vi "Cleanup.vi"(8 "error in (no error)":errorcluster, 11 "Websocket Server in":refnum<class "Websocket Server.lvclass">) -> (0 "error out":errorcluster)   [LabVIEW 2020, in "Stream-Websocket.lvlib" / "Websocket Server.lvclass"]
uses:
  Websocket Server.lvclass
  C:/dev/lv20CE/relink/lv-stream/stream/Endpoint/Endpoint.lvclass
  Websocket Server.lvclass/Websocket Server.ctl
  lv-stream/stream/Endpoint/Endpoint.lvclass
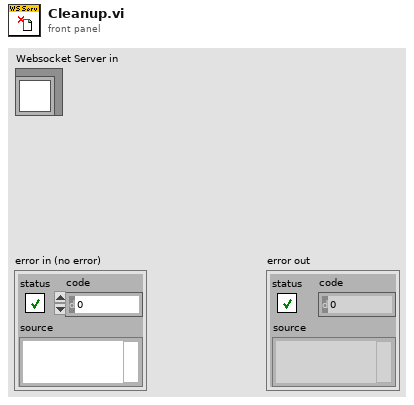
[diagram p1: front panel]
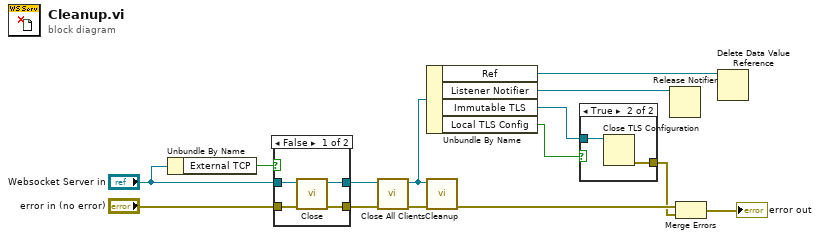
[diagram p0: block diagram]
diagram:
  n1 = Unbundle By Name("Websocket Server in") -> ("External TCP"=w2:bool)
  n2 = case shown="False" w2 {
    tunnel: "error in (no error)" -> [w18 w19]
    tunnel: [w17 w20] -> w12
    tunnel: [w16 w19] -> w11
    tunnel: "Websocket Server in" -> [w15 w20]
    frame False {
      n3 = call "Close.vi"("error in (no error)"=w18, "Endpoint in"=w15) -> ("error out"=w16:errorcluster, "Endpoint out"=w17:refnum<class "Websocket Server.lvclass">)  [unwired: 8 in]
    }
    frame True {
    }
  }
  n4 = call "Close All Clients.vi"("error in (no error)"=w11, "Websocket Server in"=w12) -> ("error out"=w10:errorcluster, "Websocket Server out"=w9:refnum<class "Websocket Server.lvclass">)  [unwired: 7 in, 1 out]
  n5 = Unbundle By Name(w9) -> ("Ref"=w7:refnum<data-value>, "Listener Notifier"=w8:refnum<notifier>, "Immutable TLS"=w4:refnum<k36>, "Local TLS Config"=w1:bool)
  n6 = call-parent "Cleanup.vi"("error in (no error)"=w10, "Endpoint in"=w9) -> ("error out"=w14:errorcluster)  [unwired: 9 in]
  n7 = case shown="True" w1 {
    tunnel: w4 -> [_ w22]
    tunnel: [_ w21] -> w5
    frame False {
    }
    frame True {
      n8 = Close TLS Configuration(11:w22) -> (0:w21:errorcluster)  [unwired: 1 in]
    }
  }
  n9 = Release Notifier(notifier=w8) -> ()  [unwired: 2 in, 3 out]
  n10 = Merge Errors(w14, w5) -> (→"error out":errorcluster)
  n11 = Delete Data Value Reference(data value reference=w7) -> ()  [unwired: 1 in, 2 out]
